vi "Load ini-file.vi"(8 "error in":errorcluster, 11 "Data Cluster in":T1) -> (0 "error out":errorcluster, 3 "Data Cluster out":T1)   [LabVIEW 2014, in "DB_CONNECTOR.lvlib"]
doc: "Load the specific configuration from the ini-file."
uses:
  DB_CONNECTOR.lvlib
  Module Data--cluster.ctl
  DB-Interface/DB-Interface.lvclass
  DB-Interface/DB-MySQL/Network Config.ctl
  hse-application/hse-application.lvclass/hse-application.ctl
  <vilib>/Utility/error.llb/Error Cluster From Error Code.vi
  hse-application/hse-application__GetSingleton.vi
  <vilib>/Utility/sysdir.llb/Get System Directory.vi
  <vilib>/ErrorRing/Error Ring.xnode
  hse-configuration/hse-config-ini/hse-config-ini.lvclass
  hse-application/hse-application.lvclass
  DB-Interface/DB-MySQL/DB-MySQL.lvclass
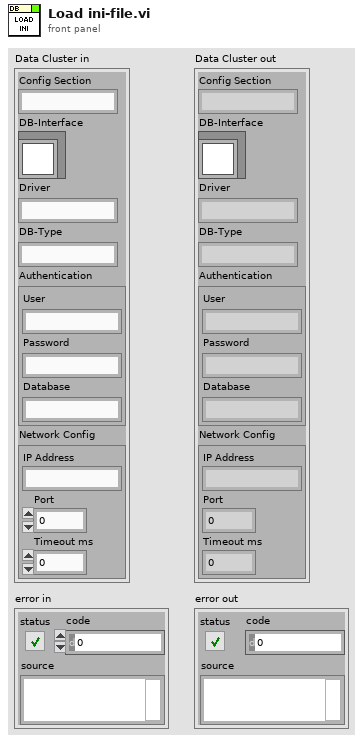
[diagram p1: front panel]
types:
  T1 = typedef "DB_CONNECTOR.lvlib/Module Data--cluster.ctl" = cluster{"Config Section":string, "DB-Interface":refnum<class "DB-Interface.lvclass">, "Driver":string, "DB-Type":string, "Authentication":cluster{"User":string, "Password":string, "Database":string}, "Network Config":T2}
  T2 = typedef "hse-db.lvlib/DB-MySQL.lvclass/Network Config.ctl" = cluster{"IP Address":string, "Port":u16, "Timeout ms":i32}
  T3 = typedef "hse-config-ini.lvclass/hse-config-ini_ConfigData.ctl" = cluster{"Path to .ini file":path}
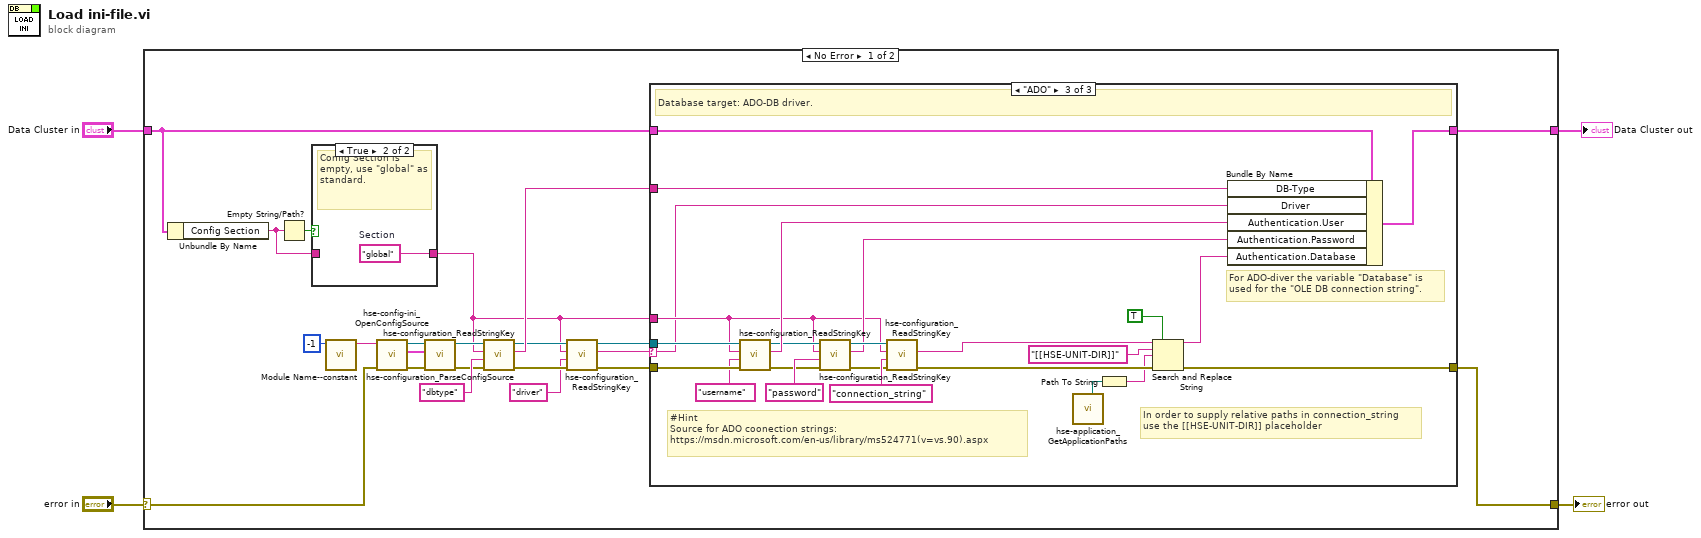
[diagram p0: block diagram]
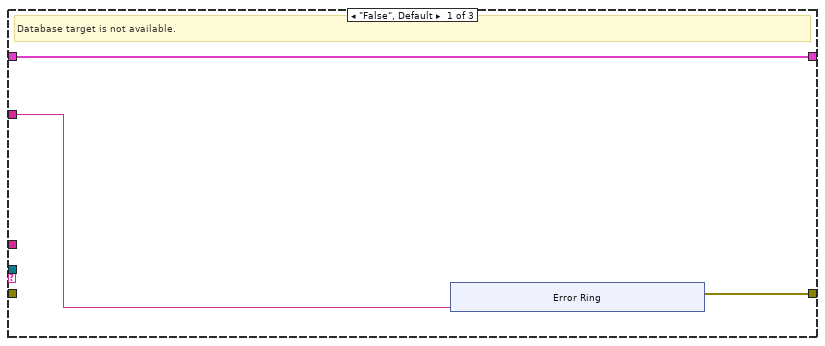
[diagram p3: hidden frame]
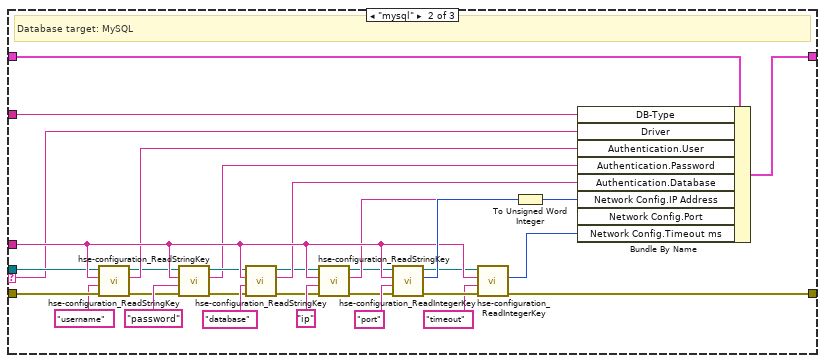
[diagram p4: hidden frame]
diagram:
  n1 = case shown="No Error" "error in" {
    selector: "error in" -> [w15 w95]
    tunnel: [w25 w95] -> w4
    tunnel: [w23 w94] -> w3
    tunnel: "Data Cluster in" -> [w13 w94]
    frame No Error {
      n2 = Unbundle By Name(w13) -> ("Config Section"=w11:string)
      n3 = Empty String/Path?(string/path=w11) -> (empty?=w12:bool)
      n4 = case shown="True" w12 {
        tunnel: w11 -> [w27 _]
        tunnel: [w27 w28] -> w7
        frame False {
          # "Config Section is given."
        }
        frame True {
          w28 = "global"  # Section
          # "Config Section is empty, use \"global\" as standard."
        }
      }
      n5 = call "Module Name--constant.vi"("Module ID"=-1) -> ("Module Name"=w16:string)  [unwired: 10 in]
      n6 = call "hse-config-ini_OpenConfigSource.vi"("error in (no error)"=w15, "Name"=w16) -> ("error out"=w17:errorcluster, "Config Data"=w19:T3, "hse-config-ini out"=w18:refnum<class "hse-config-ini.lvclass">)  [unwired: 7 in]
      n7 = call-dynamic "hse-configuration_ParseConfigSource.vi"("error in (no error)"=w17, "Config Source"=w19, "hse-config-ini in"=w18) -> ("error out"=w20:errorcluster, "hse-config-ini out"=w21:refnum<class "hse-config-ini.lvclass">)  [unwired: 7 in]
      n8 = call-dynamic "hse-configuration_ReadStringKey.vi"("error in (no error)"=w20, "Key"="dbtype", "Section"=w7, "hse-config-ini in"=w21) -> ("error out"=w24:errorcluster, "Value"=w14:string, "hse-config-ini out"=w9:refnum<class "hse-config-ini.lvclass">)  [unwired: 5 in]
      n9 = call-dynamic "hse-configuration_ReadStringKey.vi"("error in (no error)"=w24, "Key"="driver", "Section"=w7, "hse-config-ini in"=w9) -> ("error out"=w10:errorcluster, "Value"=w5:string, "hse-config-ini out"=w8:refnum<class "hse-config-ini.lvclass">)  [unwired: 5 in]
      n10 = case shown="\"ADO\"" w5 {
        selector: w5 -> [_ w39 w78]
        tunnel: [w30 w40 w74] -> w25
        tunnel: w7 -> [_ w66 w79]
        tunnel: w10 -> [_ w52 w87]
        tunnel: [w31 w49 w85] -> w23
        tunnel: w13 -> [w31 w48 w84]
        tunnel: w8 -> [_ w45 w81]
        tunnel: w14 -> [w29 w41 w80]
        frame "False", Default {
          # "Database target is not available."
          n11 = xnode "Error Ring"("parameter 0"=w29) -> ("error out"=w30:errorcluster)
        }
        frame "mysql" {
          # "Database target: MySQL"
          n12 = call-dynamic "hse-configuration_ReadStringKey.vi"("error in (no error)"=w52, "Key"="username", "Section"=w66, "hse-config-ini in"=w45) -> ("error out"=w46:errorcluster, "Value"=w53:string, "hse-config-ini out"=w47:refnum<class "hse-config-ini.lvclass">)  [unwired: 5 in]
          n13 = call-dynamic "hse-configuration_ReadStringKey.vi"("error in (no error)"=w46, "Key"="password", "Section"=w66, "hse-config-ini in"=w47) -> ("error out"=w56:errorcluster, "Value"=w55:string, "hse-config-ini out"=w57:refnum<class "hse-config-ini.lvclass">)  [unwired: 5 in]
          n14 = call-dynamic "hse-configuration_ReadStringKey.vi"("error in (no error)"=w56, "Key"="database", "Section"=w66, "hse-config-ini in"=w57) -> ("error out"=w60:errorcluster, "Value"=w59:string, "hse-config-ini out"=w44:refnum<class "hse-config-ini.lvclass">)  [unwired: 5 in]
          n15 = call-dynamic "hse-configuration_ReadStringKey.vi"("error in (no error)"=w60, "Key"="ip", "Section"=w66, "hse-config-ini in"=w44) -> ("error out"=w63:errorcluster, "Value"=w62:string, "hse-config-ini out"=w43:refnum<class "hse-config-ini.lvclass">)  [unwired: 5 in]
          n16 = call-dynamic "hse-configuration_ReadIntegerKey.vi"("error in (no error)"=w63, "Key"="port", "Section"=w66, "hse-config-ini in"=w43) -> ("error out"=w64:errorcluster, "Value"=w67:i32, "hse-config-ini out"=w42:refnum<class "hse-config-ini.lvclass">)  [unwired: 5 in]
          n17 = call-dynamic "hse-configuration_ReadIntegerKey.vi"("error in (no error)"=w64, "Key"="timeout", "Section"=w66, "hse-config-ini in"=w42) -> ("error out"=w40:errorcluster, "Value"=w68:i32)  [unwired: 5 in, 1 out]
          n18 = To Unsigned Word Integer(number=w67) -> (unsigned 16bit integer=w69:u16)
          n19 = Bundle By Name(cluster=w48, "DB-Type"=w41, "Driver"=w39, "Authentication.User"=w53, "Authentication.Password"=w55, "Authentication.Database"=w59, "Network Config.IP Address"=w62, "Network Config.Port"=w69, "Network Config.Timeout ms"=w68) -> (w49:T1)
        }
        frame "ADO" {
          # "In order to supply relative paths in connection_string\nuse the [[HSE-UNIT-DIR]] placeholder"
          # "For ADO-diver the variable \"Database\" is\nused for the \"OLE DB connection string\"."
          # "#Hint\nSource for ADO coonection strings:\nhttps://msdn.microsoft.com/en-us/library/ms524771(v=vs.90).aspx"
          # "Database target: ADO-DB driver."
          n20 = call-dynamic "hse-configuration_ReadStringKey.vi"("error in (no error)"=w87, "Key"="username", "Section"=w79, "hse-config-ini in"=w81) -> ("error out"=w82:errorcluster, "Value"=w88:string, "hse-config-ini out"=w83:refnum<class "hse-config-ini.lvclass">)  [unwired: 5 in]
          n21 = call-dynamic "hse-configuration_ReadStringKey.vi"("error in (no error)"=w82, "Key"="password", "Section"=w79, "hse-config-ini in"=w83) -> ("error out"=w91:errorcluster, "Value"=w90:string, "hse-config-ini out"=w92:refnum<class "hse-config-ini.lvclass">)  [unwired: 5 in]
          n22 = call-dynamic "hse-configuration_ReadStringKey.vi"("error in (no error)"=w91, "Key"="connection_string", "Section"=w79, "hse-config-ini in"=w92) -> ("error out"=w75:errorcluster, "Value"=w77:string)  [unwired: 5 in, 1 out]
          n23 = call "hse-application_GetApplicationPaths.vi"() -> ("Config/Unit Directory"=w71:path)  [unwired: 5 in, 6 out]
          n24 = Path To String(path=w71) -> (string=w70:string)
          n25 = Search and Replace String(replace all?=TRUE ("replace all? (F)"), input string=w77, search string="[[HSE-UNIT-DIR]]" ("Key"), replace string=w70, error in=w75) -> (result string=w76:string, error out=w74:errorcluster)  [unwired: 3 in, 2 out]
          n26 = Bundle By Name(cluster=w84, "DB-Type"=w80, "Driver"=w78, "Authentication.User"=w88, "Authentication.Password"=w90, "Authentication.Database"=w76) -> (w85:T1)
        }
      }
    }
    frame Error {
    }
  }
  "error out" <- w4
  "Data Cluster out" <- w3
